vi "Pub.vi"(1 "Data":string=" Message", 2 "Topic":string="a/b", 3 "Pub":T1) -> (0 "Error":string)   [LabVIEW 2014]
uses:
  <vilib>/addons/zeromq/zmq_socket.lvclass
  <vilib>/addons/zeromq/zmq_context.lvclass
  <vilib>/daq.io/MQTT LabVIEW Client/Controls/QoS.ctl
  <vilib>/daq.io/MQTT LabVIEW Client/Controls/Retain_Flag.ctl
  <vilib>/daq.io/MQTT LabVIEW Client/Controls/DUP_Flag.ctl
  Pub.global.vi
  <vilib>/daq.io/MQTT LabVIEW Client/MQTT_Functions.lvlib
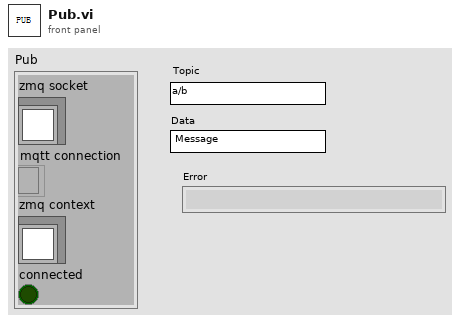
[diagram p1: front panel]
types:
  T1 = cluster{"zmq socket":refnum<class "zmq_socket.lvclass">, "mqtt connection":refnum<k5>, "zmq context":refnum<class "zmq_context.lvclass">, "connected":bool}
  T2 = typedef "MQTT_Functions.lvlib/QoS.ctl" = enum8{"At most once", "At least once", "Exactly once", "Reserved"}
  T3 = typedef "MQTT_Functions.lvlib/Retain_Flag.ctl" = bool
  T4 = typedef "MQTT_Functions.lvlib/DUP_Flag.ctl" = bool
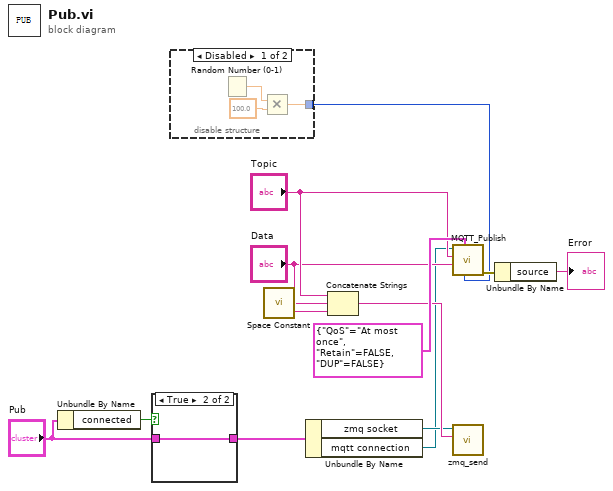
[diagram p0: block diagram]
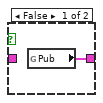
[diagram p2: hidden frame]
diagram:
  n1 = Unbundle By Name("Pub") -> ("connected"=w5:bool)
  n2 = case shown="True" w5 {
    tunnel: "Pub" -> [_ w15]
    tunnel: [w14 w15] -> w3
    frame False {
      n3 = global read "Pub.global.vi" "Pub"() -> (w14:T1)
    }
    frame True {
    }
  }
  n4 = disable-structure shown="Disabled" {
    disable-tunnel: [w18 _] -> w11
    frame Disabled {
      n5 = Random Number (0-1)() -> (number: 0 to 1=w16:dbl)
      n6 = Multiply(x=w16, y=100.0) -> (x*y=w18:dbl)
    }
    frame Enabled {
    }
  }
  n7 = call <vilib>:"Space Constant.vi"() -> ("String"=w7:string)
  n8 = Unbundle By Name(w3) -> ("zmq socket"=w2:refnum<class "zmq_socket.lvclass">, "mqtt connection"=w1:refnum<k5>)
  n9 = Concatenate Strings("Topic", w7, "Data") -> (w6:string)
  n10 = call <vilib>:"MQTT_Publish.vi"("Message ID"=w11, "Publish Meta"=cluster{"QoS":T2, "Retain":T3, "DUP":T4} {"QoS"=enum."At most once", "Retain"=FALSE, "DUP"=FALSE}, "Message to be published"="Data", "Topic"="Topic", "connection ID"=w1) -> ("error out"=w12:errorcluster)  [unwired: 5 in, 1 out]
  n11 = call <vilib>:"zmq_send.vi"("data"=w6, "socket in"=w2) -> ()  [unwired: 5 in, 2 out]
  n12 = Unbundle By Name(w12) -> ("source"=→"Error":string)
